vi "HostSequencerSimpleTest.vi"() -> ()   [LabVIEW 2014]
uses:
  <vilib>/FPGAPlugInAG/PXI-7852R/niLvFpga_Open_PXI-7852R.vi
  <vilib>/rvi/interface/common/dynamic/niFpgaDynamicAddResources.vi
  <vilib>/Utility/error.llb/Error Cluster From Error Code.vi
  <vilib>/rvi/errors/niLvFpgaAdjustHostInterfaceError.vi
  <vilib>/FPGAPlugInAG/Dynamic/niLvFpga_Close_Dynamic.vi
  <vilib>/rvi/interface/nirviOpenFPGA/nirviOpenFPGA.xnode
  FPGA Bitfiles/TiTaProj_DAF_sequencerTopLeve_WBop0GaikJk.lvbitx
  sequencerTopLevel.vi
  <vilib>/rvi/interface/nirviReadWriteControl/nirviReadWriteControl.xnode
  <vilib>/rvi/interface/nirviMethod/nirviMethod.xnode
  <vilib>/rvi/interface/nirviCloseFPGA/nirviCloseFPGA.xnode
  <vilib>/FPGAPlugInAG/Dynamic/niLvFpga_WriteFifo_Dynamic.vi
  <vilib>/rvi/errors/niLvFpgaMergeErrorWithErrorCode.vi
  NiFpgaLv.dll
  <vilib>/rvi/interface/Simulation/niFpgaSimulationCallBeginRW.vi
panel:
  out "Empty Elements Remaining":u32
  in  "Timeout (ms)":i32=5000
  in  "start":bool
  in  "stop":bool
  out "timeOutSetVolt":bool
  out "Scanning":bool
  in  "nOfScanRegions":i32
  in  "Data":u32[](array[numeric]) format="%024b"
  in  "waitForKepco /t":u32
  in  "nOfCycles":i32
  in  "nOfLoops":i32
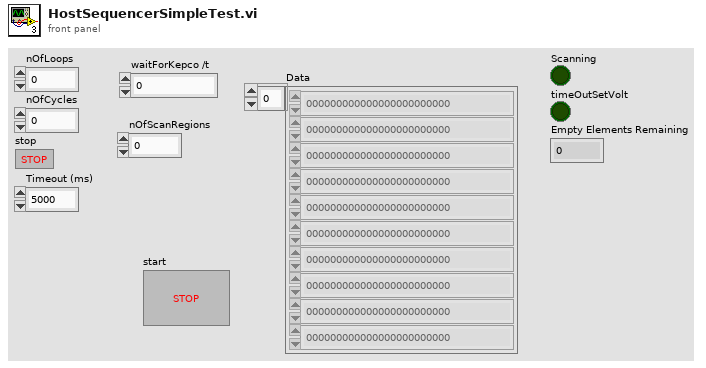
[diagram p1: front panel]
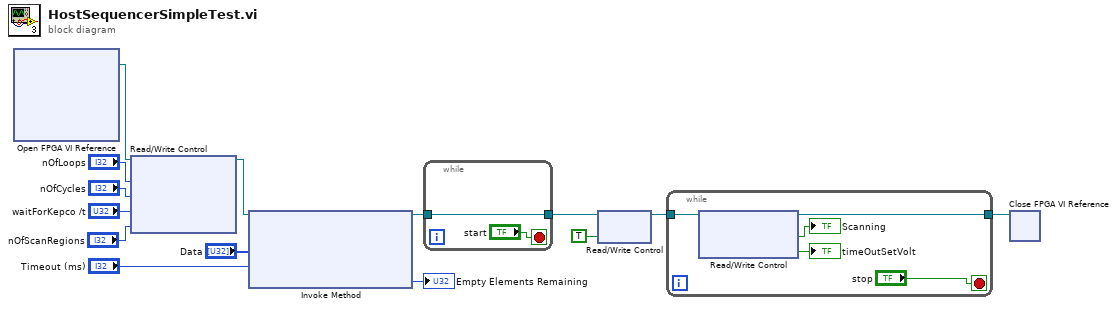
[diagram p0: block diagram]
diagram:
  n1 = xnode ("Open FPGA VI Reference")() -> ("FPGA VI Reference Out"=w14:refnum<k20>)  [unwired: 2 in, 1 out]
  n2 = xnode "Read/Write Control"("FPGA VI Reference In"=w14, "nOfLoops"="nOfLoops", "nOfCycles"="nOfCycles", "waitForKepco /t"="waitForKepco /t", "nOfScanRegions"="nOfScanRegions") -> ("FPGA VI Reference Out"=w10:refnum<k20>)  [unwired: 1 in, 1 out]
  n3 = xnode "Invoke Method"("FPGA VI Reference In"=w10, "Data"="Data", "Timeout (ms)"="Timeout (ms)") -> ("FPGA VI Reference Out"=w5:refnum<k20>, "Empty Elements Remaining"=→"Empty Elements Remaining":u32)  [unwired: 1 in, 1 out]
  n4 = while {
    tunnel: w5 -> [w16]
    tunnel: [w16] -> w4
    stop <- "start" stop-if-true
  }
  n5 = xnode "Read/Write Control"("FPGA VI Reference In"=w4, "start"=TRUE) -> ("FPGA VI Reference Out"=w6:refnum<k20>)  [unwired: 1 in, 1 out]
  n6 = while {
    tunnel: w6 -> [w21]
    tunnel: [w17] -> w7
    stop <- "stop" stop-if-true
    n7 = xnode "Read/Write Control"("FPGA VI Reference In"=w21) -> ("FPGA VI Reference Out"=w17:refnum<k20>, "Scanning"=→"Scanning":bool, "timeOutSetVolt"=→"timeOutSetVolt":bool)  [unwired: 1 in, 1 out]
  }
  n8 = xnode "Close FPGA VI Reference"("FPGA VI Reference In"=w7) -> ()  [unwired: 1 in, 1 out]
